vi "提取日志报警参数入列队 (子VI).vi"(10 "索引":i32, 11 "队列输入":refnum<queue>) -> ()   [LabVIEW 2016, in "数据传输系统.lvlib"]
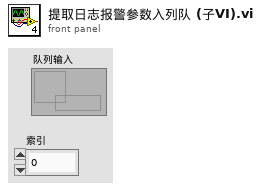
[diagram p1: front panel]
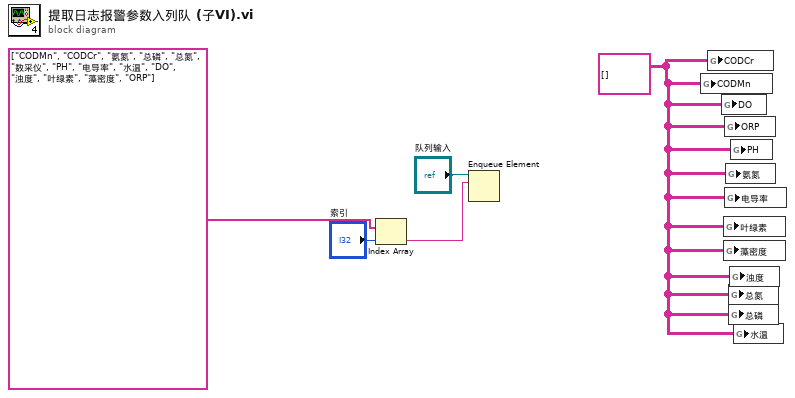
[diagram p0: block diagram]
diagram:
  w1 = string[][] [] ("氨氮")
  n1 = Index Array(array=string[] ["CODMn", "CODCr", "氨氮", "总磷", "总氮", "数采仪", "PH", "电导率", "水温", "DO", "浊度", "叶绿素", "藻密度", "ORP"], index="索引") -> (element=w3:string)
  n2 = Enqueue Element(queue="队列输入", element=w3) -> ()  [unwired: 2 in, 3 out]
  n3 = global write "全局 所有参数.vi" "CODMn"(w1) -> ()
  n4 = global write "全局 所有参数.vi" "CODCr"(w1) -> ()
  n5 = global write "全局 所有参数.vi" "DO"(w1) -> ()
  n6 = global write "全局 所有参数.vi" "叶绿素"(w1) -> ()
  n7 = global write "全局 所有参数.vi" "藻密度"(w1) -> ()
  n8 = global write "全局 所有参数.vi" "ORP"(w1) -> ()
  n9 = global write "全局 所有参数.vi" "电导率"(w1) -> ()
  n10 = global write "全局 所有参数.vi" "氨氮"(w1) -> ()
  n11 = global write "全局 所有参数.vi" "总氮"(w1) -> ()
  n12 = global write "全局 所有参数.vi" "总磷"(w1) -> ()
  n13 = global write "全局 所有参数.vi" "浊度"(w1) -> ()
  n14 = global write "全局 所有参数.vi" "PH"(w1) -> ()
  n15 = global write "全局 所有参数.vi" "水温"(w1) -> ()
